vi "CCE T027 SubVI04.vi"(9 "q":dbl, 10 "p":dbl, 11 "Image Data":u8[][](array[numeric])) -> (3 "MC":dbl)   [LabVIEW 2020]
doc: "Ceballos Conde Emanuel 4MV6 Sistemas de visión artificial 2022/1\neste vi permite obtener el momento central"
panel:
  # "Ceballos Conde Emanuel\n4MV6\nSistemas de visión artificial\n2022/1"
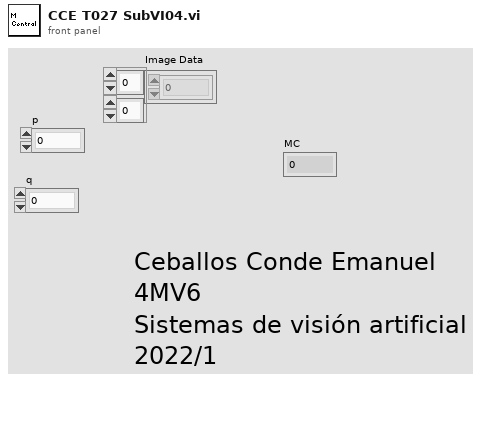
[diagram p1: front panel]
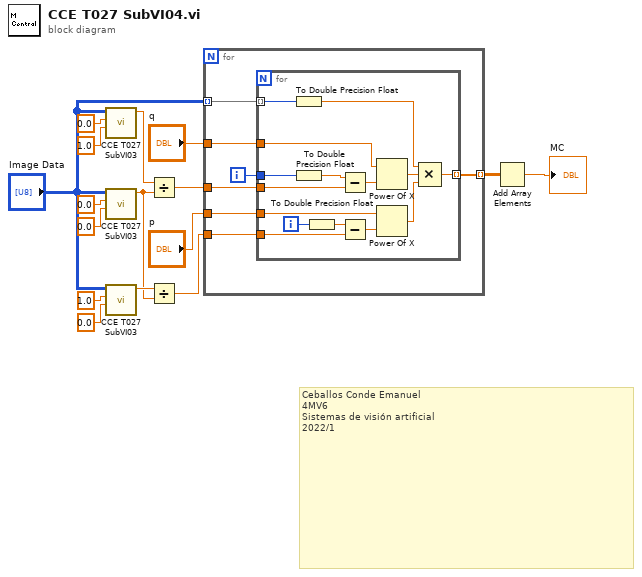
[diagram p0: block diagram]
diagram:
  # "Ceballos Conde Emanuel\n4MV6\nSistemas de visión artificial\n2022/1"
  n1 = call "CCE T027 SubVI03.vi"("q"=1.0, "p"=0.0, "Image Data"="Image Data") -> ("M. Inicial"=w9:dbl)  [unwired: 8 in]
  n2 = call "CCE T027 SubVI03.vi"("q"=0.0, "p"=0.0, "Image Data"="Image Data") -> ("M. Inicial"=w8:dbl)  [unwired: 8 in]
  n3 = call "CCE T027 SubVI03.vi"("q"=0.0, "p"=1.0, "Image Data"="Image Data") -> ("M. Inicial"=w10:dbl)  [unwired: 8 in]
  n4 = Divide(x=w9, y=w8) -> (x/y=w2:dbl)
  n5 = Divide(x=w10, y=w8) -> (x/y=w1:dbl)
  n6 = for {
    tunnel: "Image Data" -> [w23] mode=indexing
    tunnel: "q" -> [w22]
    tunnel: "p" -> [w21]
    tunnel: [w19] -> w7 mode=indexing
    tunnel: w2 -> [w18]
    tunnel: w1 -> [w17]
    i -> [w20]
    n7 = for {
      tunnel: w23 -> [w34] mode=indexing
      tunnel: w22 -> [w38]
      tunnel: w21 -> [w37]
      tunnel: w20 -> [w32]
      tunnel: [w30] -> w19 mode=indexing
      tunnel: w18 -> [w27]
      tunnel: w17 -> [w24]
      i -> [w33]
      n8 = To Double Precision Float(number=w34) -> (double precision float=w31:dbl)
      n9 = To Double Precision Float(number=w32) -> (double precision float=w29:dbl)
      n10 = To Double Precision Float(number=w33) -> (double precision float=w25:dbl)
      n11 = Subtract(x=w29, y=w27) -> (x-y=w28:dbl)
      n12 = Subtract(x=w25, y=w24) -> (x-y=w26:dbl)
      n13 = Power Of X(1:w28, 2:w38) -> (0:w36:dbl)
      n14 = Power Of X(1:w26, 2:w37) -> (0:w35:dbl)
      n15 = Compound Arithmetic op=MULTIPLY(w31, w36, w35) -> (w30:dbl)
    }
  }
  n16 = Add Array Elements(numeric array=w7) -> (sum=→"MC":dbl)
